vi "DAQ Assist_AD_DA.vi"() -> ()   [LabVIEW 2010]
panel:
  in  "stop 2":bool
  in  "stop":bool
  in  "Boolean":bool
  out "Waveform Graph 2":dynamicdata(graph)
  in  "error in 2":errorcluster caption="error in"
  out "迴圈時間ms":u32 format="%.6f"
  # "擷取卡通道\nAO6\nAO7\n\nAI1\nAI7"
  # "連續取樣"
  # "N sample"
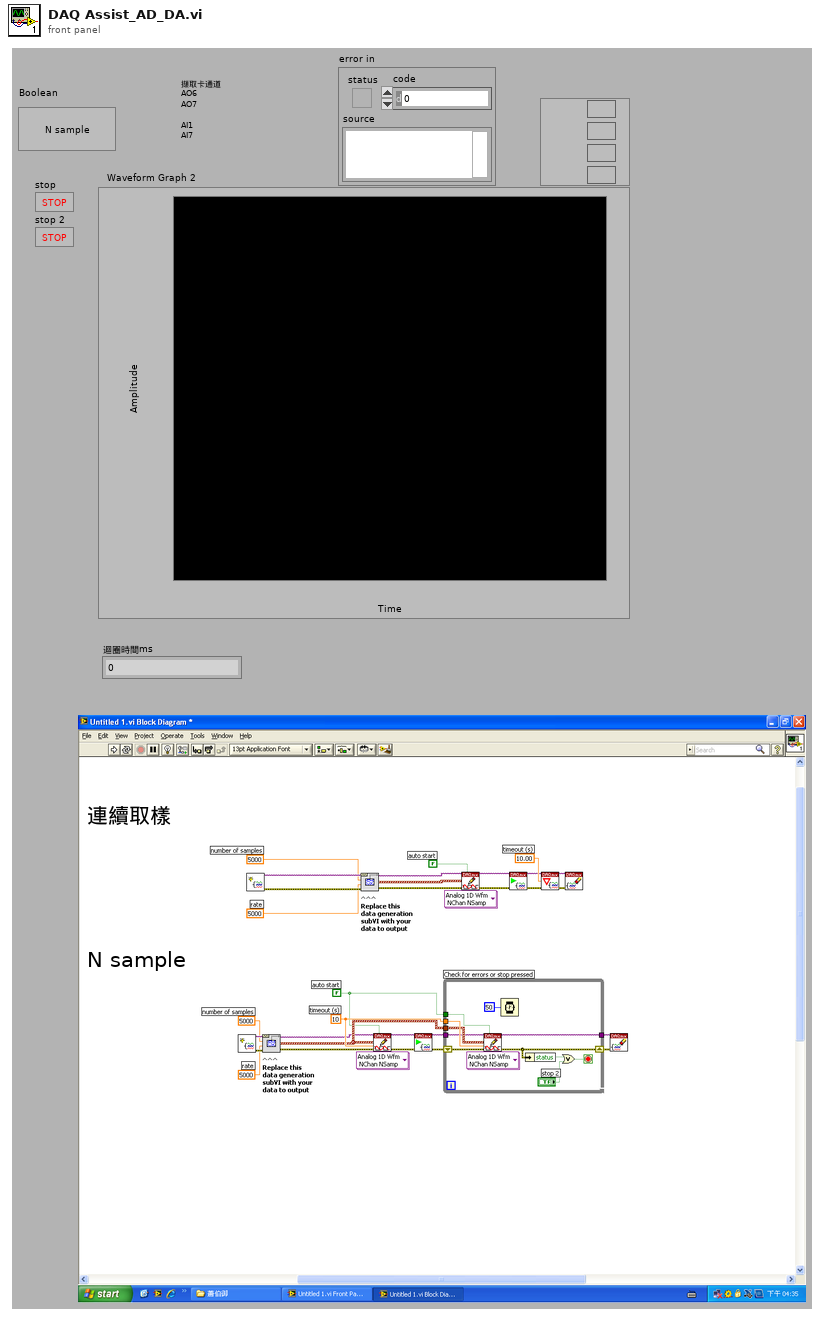
[diagram p1: front panel]
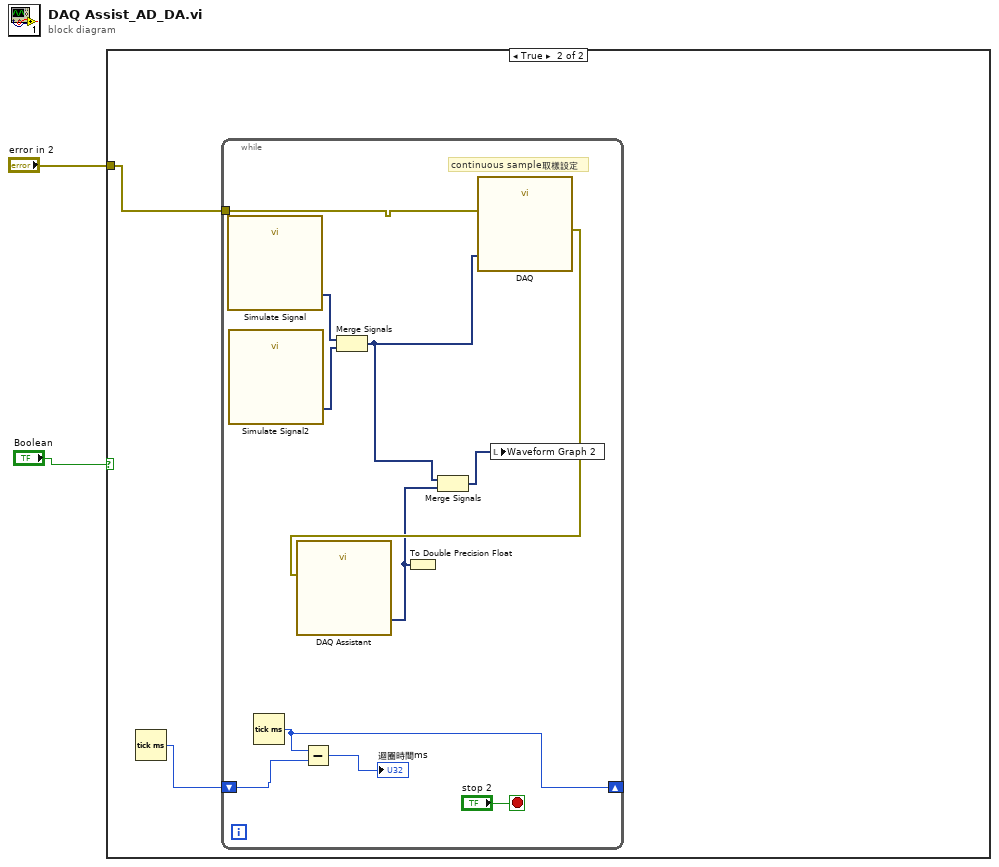
[diagram p0: block diagram]
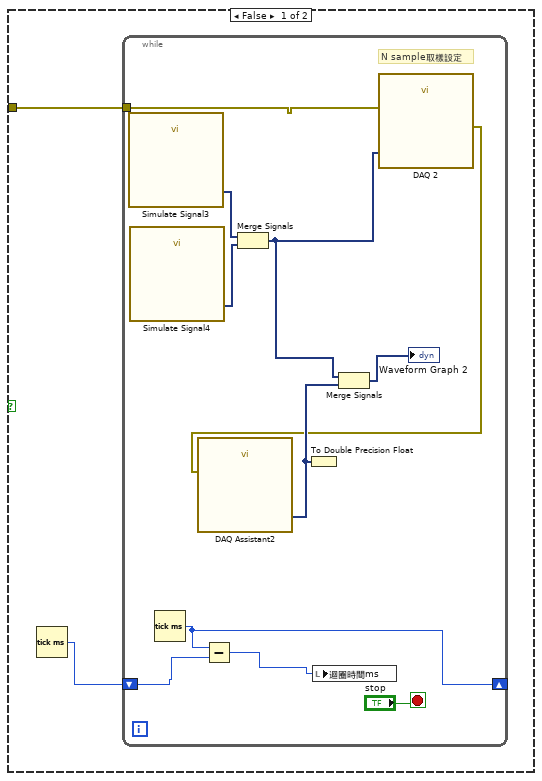
[diagram p2: hidden frame]
diagram:
  n1 = case shown="True" "Boolean" {
    tunnel: "error in 2" -> [w3 w16]
    frame False {
      n2 = Tick Count (ms)() -> (millisecond timer value=w4:u32)
      n3 = while {
        shift-right: [w14] -> _
        shift-left: w4 -> [w15]
        tunnel: w3 -> [w6]
        stop <- "stop" stop-if-true
        # "N sample取樣設定"
        n4 = call "Simulate Signal3"() -> ("Sine"=w13:dynamicdata)  [unwired: 14 in, 1 out]
        n5 = call "Simulate Signal4"() -> ("Sine"=w12:dynamicdata)  [unwired: 14 in, 1 out]
        n6 = Tick Count (ms)() -> (millisecond timer value=w14:u32)
        n7 = Subtract(x=w14, y=w15) -> (x-y=w7:u32)
        n8 = Merge Signals(w13, w12) -> (w9:dynamicdata)
        n9 = local write "迴圈時間ms"(w7) -> ()
        n10 = call "DAQ 2"("data"=w9, "error in"=w6) -> ("error out"=w8:errorcluster)  [unwired: 16 in, 1 out]
        n11 = call "DAQ Assistant2"("error in"=w8) -> ("data"=w11:dynamicdata)  [unwired: 15 in, 3 out]
        n12 = To Double Precision Float(number=w11) -> ()  [unwired: 1 out]
        n13 = Merge Signals(w9, w11) -> (→"Waveform Graph 2":dynamicdata)
      }
    }
    frame True {
      n14 = Tick Count (ms)() -> (millisecond timer value=w17:u32)
      n15 = while {
        shift-right: [w27] -> _
        shift-left: w17 -> [w28]
        tunnel: w16 -> [w19]
        stop <- "stop 2" stop-if-true
        # "continuous sample取樣設定"
        n16 = call "Simulate Signal"() -> ("Sine"=w25:dynamicdata)  [unwired: 14 in, 1 out]
        n17 = call "Simulate Signal2"() -> ("Sine"=w24:dynamicdata)  [unwired: 14 in, 1 out]
        n18 = Tick Count (ms)() -> (millisecond timer value=w27:u32)
        n19 = Subtract(x=w27, y=w28) -> (x-y=→"迴圈時間ms":u32)
        n20 = Merge Signals(w25, w24) -> (w23:dynamicdata)
        n21 = call "DAQ"("data"=w23, "error in"=w19) -> ("error out"=w22:errorcluster)  [unwired: 15 in, 2 out]
        n22 = call "DAQ Assistant"("error in"=w22) -> ("data"=w20:dynamicdata)  [unwired: 15 in, 3 out]
        n23 = To Double Precision Float(number=w20) -> ()  [unwired: 1 out]
        n24 = Merge Signals(w23, w20) -> (w21:dynamicdata)
        n25 = local write "Waveform Graph 2"(w21) -> ()
      }
    }
  }
